vi "4.1.vi"() -> ()   [LabVIEW 2017]
panel:
  out "波形图":cluster{i32, i32, dbl[]}[](graph)
  # "任务一"
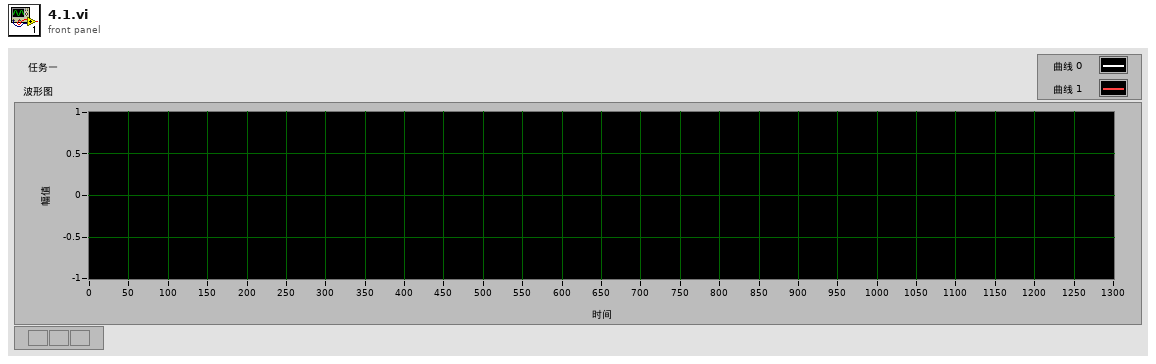
[diagram p1: front panel]
types:
  T1 = cluster{cluster{i32, i32, dbl[]}, cluster{i32, i32, dbl[]}}
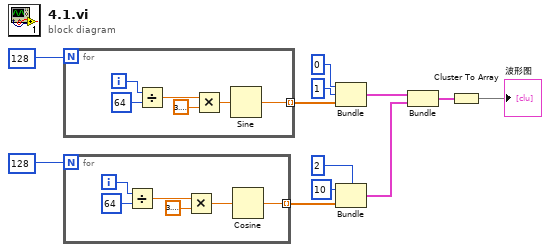
[diagram p0: block diagram]
diagram:
  n1 = for {
    N: 128 -> [_]
    tunnel: [w18] -> w11 mode=indexing
    i -> [w14]
    n2 = Divide(x=w14, y=64) -> (x/y=w16:dbl)
    n3 = Multiply(x=w16, y=3.141592653589793) -> (x*y=w13:dbl)
    n4 = Sine(x=w13) -> (sin(x)=w18:dbl)
  }
  n5 = for {
    N: 128 -> [_]
    tunnel: [w24] -> w7 mode=indexing
    i -> [w19]
    n6 = Divide(x=w19, y=64) -> (x/y=w22:dbl)
    n7 = Multiply(x=w22, y=3.141592653589793) -> (x*y=w20:dbl)
    n8 = Cosine(x=w20) -> (cos(x)=w24:dbl)
  }
  n9 = Bundle(0, 1, w11) -> (w3:cluster{i32, i32, dbl[]})  [unwired: 1 in]
  n10 = Bundle(2, 10, w7) -> (w4:cluster{i32, i32, dbl[]})  [unwired: 1 in]
  n11 = Bundle(w3, w4) -> (w2:T1)  [unwired: 1 in]
  n12 = Cluster To Array(cluster=w2) -> (array=→"波形图":cluster{i32, i32, dbl[]}[])
